vi "p1.vi"() -> ()   [LabVIEW 2021, in "d12.lvlib"]
uses:
  d12.lvlib
  AOC/AOC.lvlib
panel:
  out "Route":cluster{"row":i32, "col":i32}[](graph)
  out "Height Map":i16[][](graph)
  out "Answer":i32
  in  "Example":string="Sabqponm\nabcryxxl\naccszExk\nacctuvwj\nabdefghi"
  in  "Example":bool
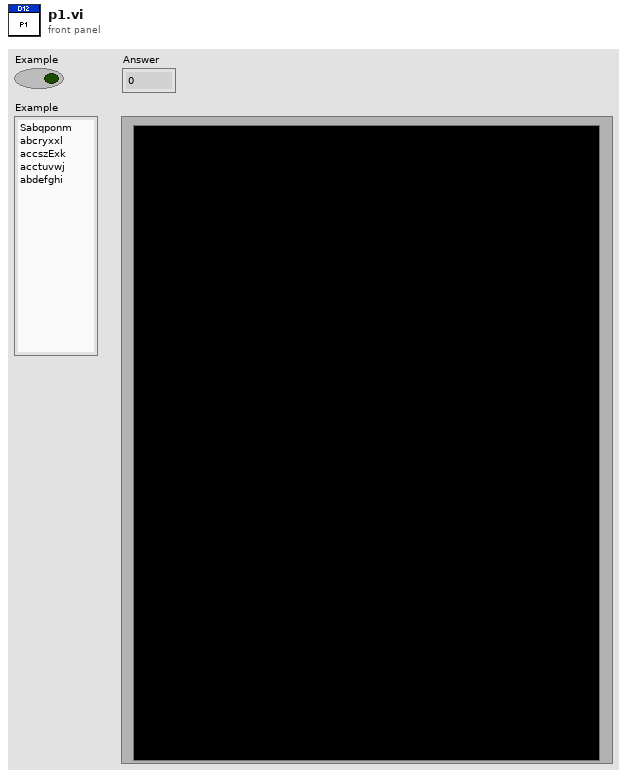
[diagram p1: front panel]
types:
  T1 = map{cluster{"row":i32, "col":i32}, cluster{"Height":i16, "Parent":cluster{"row":i32, "col":i32}, "Explored?":bool}}
  T2 = cluster{"Height":i16, "Parent":cluster{"row":i32, "col":i32}, "Explored?":bool}
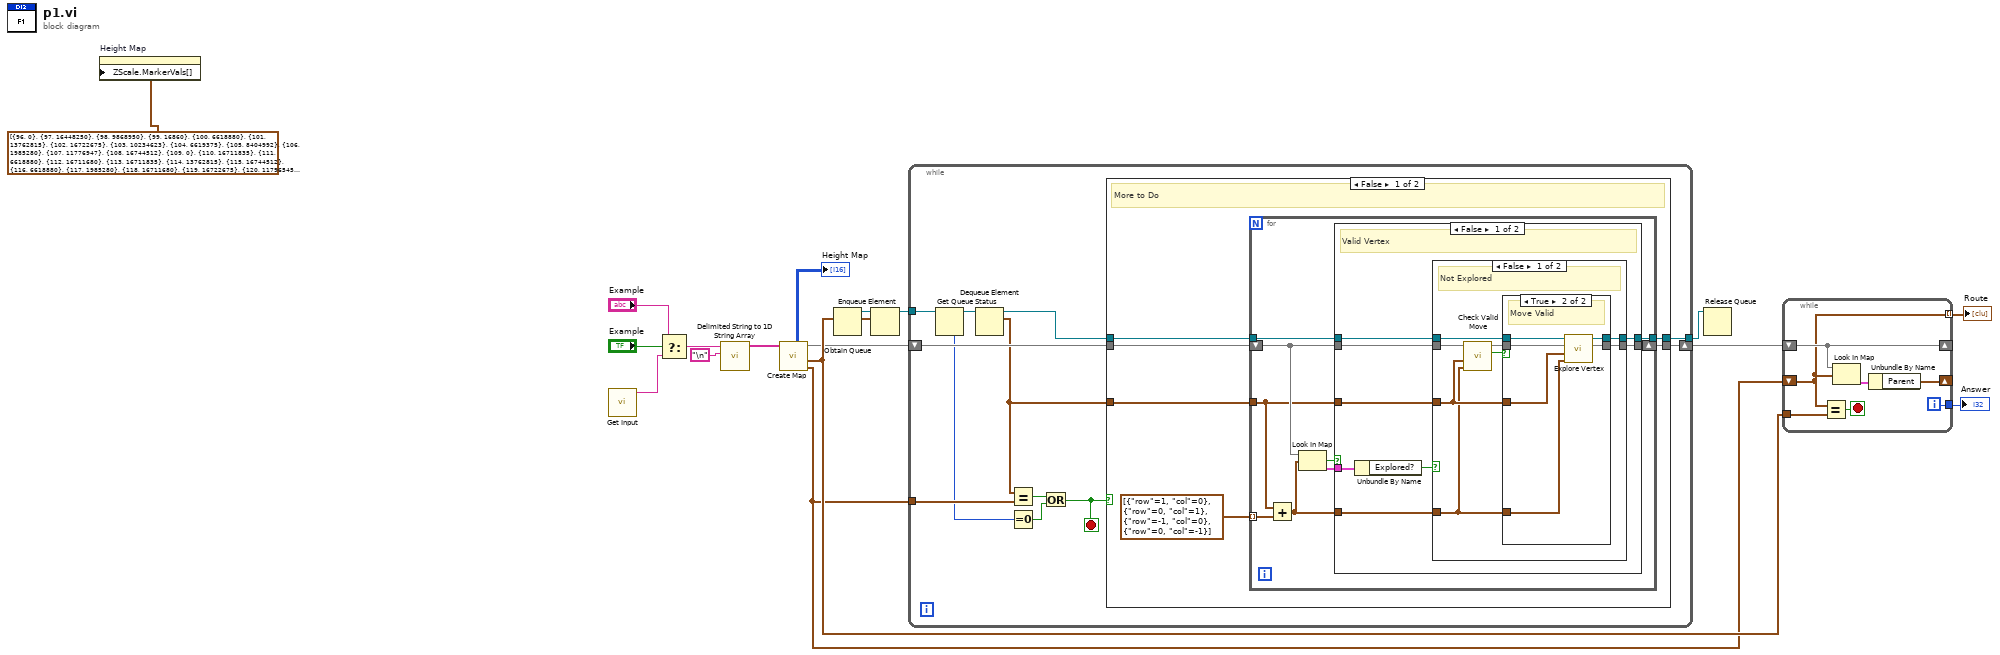
[diagram p0: block diagram]
diagram:
  n1 = property on="Height Map" class="IntGraph (strict)"("ZScale.MarkerVals[]"=cluster{i16, u32}[] [{96, 0}, {97, 16448250}, {98, 9868950}, {99, 16860}, {100, 6618880}, {101, 13762815}, {102, 16722675}, {103, 10234623}, {104, 6619375}, {105, 8404992}, {106, 1985280}, {107, 11776947}, {108, 16744512}, {109, 0}, {110, 16711835}, {111, 6618880}, {112, 16711680}, {113, 16711835}, {114, 13762815}, {115, 16744512}, {116, 6618880}, {117, 1985280}, {118, 16711680}, {119, 16722675}, {120, 11796545}, {121, 7171459}, {122, 7171459}, {123, 0}] ("Z Scale.Marker Values[]")) -> ()  [unwired: 2 in, 2 out]
  n2 = call "Get Input.vi"() -> ("Input"=w17:string)  [unwired: 11 in]
  n3 = Select(t="Example", s="Example", f=w17) -> (s? t:f=w16:string)
  n4 = call <vilib>:"Delimited String to 1D String Array.vi"("delimiter"="\n", "delimited string"=w16) -> ("string array"=w12:string[])  [unwired: 9 in]
  n5 = call "Create Map.vi"("input"=w12) -> ("End"=w3:cluster{"row":i32, "col":i32}, "Start"=w8:cluster{"row":i32, "col":i32}, "Map"=w5:T1, "Heights"=→"Height Map":i16[][])  [unwired: 7 in]
  n6 = Obtain Queue(element data type=w8) -> (queue out=w11:refnum<queue>)  [unwired: 4 in, 2 out]
  n7 = Enqueue Element(queue=w11, element=w8) -> (queue out=w10:refnum<queue>)  [unwired: 2 in, 2 out]
  n8 = while {
    shift-right: [w26] -> w9
    shift-left: w5 -> [w29]
    tunnel: w3 -> [w28]
    tunnel: w10 -> [w22]
    tunnel: [w18] -> w2
    stop <- w20 stop-if-true
    n9 = Get Queue Status(queue=w22) -> (queue out=w23:refnum<queue>, # elements in queue=w21:i32)  [unwired: 2 in, 6 out]
    n10 = Dequeue Element(queue=w23) -> (queue out=w24:refnum<queue>, element=w25:cluster{"row":i32, "col":i32})  [unwired: 2 in, 2 out]
    n11 = Equal?(x=w25, y=w28) -> (x = y?=w27:bool)
    n12 = Equal To 0?(x=w21) -> (x = 0?=w19:bool)
    n13 = Or(x=w27, y=w19) -> (x .or. y?=w20:bool)
    n14 = case shown="False" w20 {
      tunnel: w29 -> [w32 w74]
      tunnel: w25 -> [w31 _]
      tunnel: [w35 w74] -> w26
      tunnel: w24 -> [w33 w73]
      tunnel: [w30 w73] -> w18
      frame False {
        # "More to Do"
        n15 = for {
          tunnel: w31 -> [w36]
          shift-right: [w41] -> w35
          shift-left: w32 -> [w42]
          tunnel: cluster{"row":i32, "col":i32}[] [{"row"=1, "col"=0}, {"row"=0, "col"=1}, {"row"=-1, "col"=0}, {"row"=0, "col"=-1}] ("element") -> [w44] mode=indexing
          tunnel: w33 -> [w39]
          tunnel: [w37] -> w30
          n16 = Add(x=w36, y=w44) -> (x+y=w38:cluster{"row":i32, "col":i32})
          n17 = Look In Map(map=w42, key=w38) -> (key not found?=w43:bool, value=w40:T2)  [unwired: 1 in]
          n18 = case shown="False" w43 {
            tunnel: w42 -> [w47 w72]
            tunnel: [w46 w72] -> w41
            tunnel: w40 -> [w51 _]
            tunnel: w39 -> [w48 w71]
            tunnel: w36 -> [w50 _]
            tunnel: w38 -> [w49 _]
            tunnel: [w45 w71] -> w37
            frame False {
              # "Valid Vertex"
              n19 = Unbundle By Name(w51) -> ("Explored?"=w52:bool)
              n20 = case shown="False" w52 {
                tunnel: w50 -> [w57 _]
                tunnel: w49 -> [w56 _]
                tunnel: w48 -> [w60 w69]
                tunnel: w47 -> [w53 w70]
                tunnel: [w59 w70] -> w46
                tunnel: [w58 w69] -> w45
                frame False {
                  # "Not Explored"
                  n21 = call "Check Valid Move.vi"("Vertex"=w56, "Parent"=w57, "Map in"=w53) -> ("Valid Move?"=w55:bool, "Map out"=w54:T1)  [unwired: 7 in]
                  n22 = case shown="True" w55 {
                    tunnel: w57 -> [_ w68]
                    tunnel: w60 -> [w61 w67]
                    tunnel: w56 -> [_ w63]
                    tunnel: w54 -> [w62 w66]
                    tunnel: [w62 w65] -> w59
                    tunnel: [w61 w64] -> w58
                    frame False {
                      # "Move Invalid"
                    }
                    frame True {
                      # "Move Valid"
                      n23 = call "Explore Vertex.vi"("Vertex"=w63, "Parent"=w68, "Map in"=w66, "Queue in"=w67) -> ("Map out"=w65:T1, "Queue out"=w64:refnum<queue>)  [unwired: 6 in]
                    }
                  }
                }
                frame True {
                  # "Explored"
                }
              }
            }
            frame True {
              # "Invalid Vertex"
            }
          }
        }
      }
      frame True {
        # "Nothing Left to Do"
      }
    }
  }
  n24 = Release Queue(queue=w2) -> ()  [unwired: 2 in, 3 out]
  n25 = while {
    shift-right: [w81] -> _
    shift-left: w9 -> [w81]
    shift-right: [w79] -> _
    shift-left: w3 -> [w75]
    tunnel: w8 -> [w78]
    tunnel: [w76] -> w7
    tunnel: [w75] -> w1 mode=indexing
    i -> [w76]
    stop <- w77 stop-if-true
    n26 = Equal?(x=w75, y=w78) -> (x = y?=w77:bool)
    n27 = Look In Map(map=w81, key=w75) -> (value=w80:T2)  [unwired: 1 in, 1 out]
    n28 = Unbundle By Name(w80) -> ("Parent"=w79:cluster{"row":i32, "col":i32})
  }
  "Answer" <- w7
  "Route" <- w1
